vi "NF LI56xx dvr sCLS.vi"(8 "error in":errorcluster caption="error in (no error)" {"code" format="%.0x"}, 11 "VISA resource name":refnum<visa-resource-name>) -> (0 "error out":errorcluster {"code" format="%.0x"}, 3 "VISA resource name copy":refnum<visa-resource-name>)   [LabVIEW 2019]
doc: "Clears the following statuses. \n Standard Event Status register\n Operation Event register\n Questionable Event register\n Status byte\n Error queue\nAlso clears the panel error display."
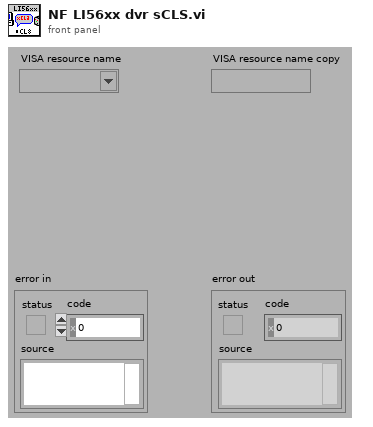
[diagram p1: front panel]
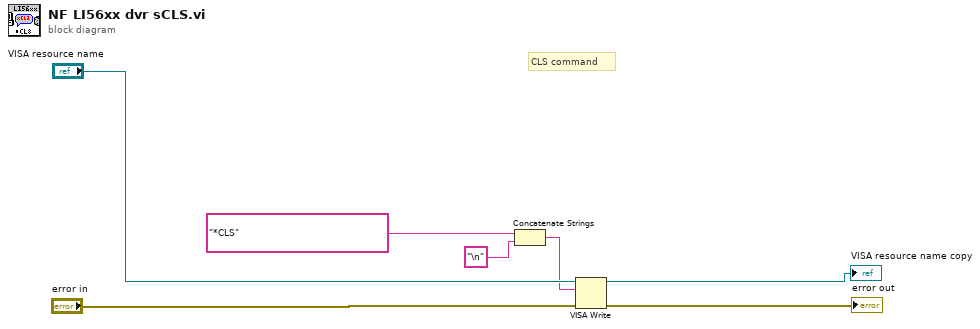
[diagram p0: block diagram]
diagram:
  # "CLS command"
  n1 = Concatenate Strings("*CLS" ("•¶Žš—ñ"), "\n" ("Œ`Ž®•¶Žš—ñ")) -> (w4:string)
  n2 = VISA Write(VISA resource name="VISA resource name", write buffer=w4, error in (no error)="error in") -> (VISA resource name out=→"VISA resource name copy":refnum<visa-resource-name>, error out=→"error out":errorcluster)  [unwired: 1 out]
